vi "Start Sync.vi"(8 "error in (no error)":errorcluster, 10 "current time":timestamp, 11 "gRPC Server in":refnum<class "HVC2.lvclass">) -> (0 "error out":errorcluster, 3 "gRPC Server out":refnum<class "HVC2.lvclass">)   [LabVIEW 2019, in "HVC2.lvlib" / "HVC2.lvclass"]
uses:
  HVC2.lvclass
  RPC Messages/measurementservice_DMMConfigRequest/measurementservice_DMMConfigRequest_Data.ctl
  HVC2.lvclass/HVC2.ctl
  RPC Messages/measurementservice_QueryResponse/measurementservice_QueryResponse_Data.ctl
  RPC Messages/measurementservice_DMMConfigResponse/measurementservice_DMMConfigResponse_Data.ctl
  RPC Messages/measurementservice_ErrorOut/measurementservice_ErrorOut_Data.ctl
  RPC Messages/measurementservice_DMMVoltageData/measurementservice_DMMVoltageData_Data.ctl
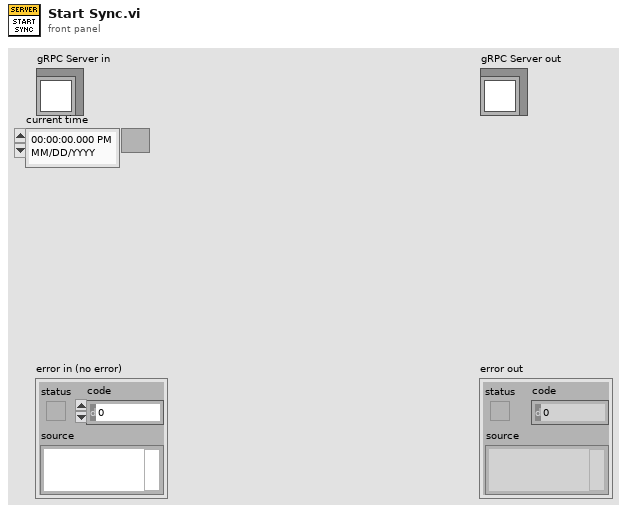
[diagram p1: front panel]
types:
  T1 = typedef "HVC2.lvlib/HVC2.lvclass/measurementservice_DMMConfigRequest_Data.ctl" = cluster{"DMMFunction":i32, "DMMResolution":sgl, "DMMRange":sgl, "DMMSampleCount":i32, "DMMApertureTimeUnit":i32, "DMMApertureTime":sgl, "DMMNumberofAverages":i32, "DMMAutoZero":i32, "DMMADCCalibration":i32, "DMMSettleTime":sgl}
  T2 = cluster{"measurementservice_DMMConfigRequest_Data":T1}
  T3 = typedef "HVC2.lvlib/HVC2.lvclass/measurementservice_QueryResponse_Data.ctl" = cluster{"message":string, "status":i32}
  T4 = typedef "HVC2.lvlib/HVC2.lvclass/measurementservice_ErrorOut_Data.ctl" = cluster{"errCode":i32, "errMessage":string}
  T5 = typedef "HVC2.lvlib/HVC2.lvclass/measurementservice_DMMConfigResponse_Data.ctl" = cluster{"DMMFunction":i32, "DMMResolution":sgl, "DMMRange":sgl, "DMMSampleCount":i32, "DMMApertureTimeUnit":i32, "DMMApertureTime":sgl, "DMMNumberofAverages":i32, "DMMAutoZero":i32, "DMMADCCalibration":i32, "DMMSettleTime":sgl, "error":T4}
  T6 = typedef "HVC2.lvlib/HVC2.lvclass/measurementservice_DMMVoltageData_Data.ctl" = cluster{"voltage":sgl, "error":T4}
  T7 = typedef "HVC2.lvlib/HVC2.lvclass/Server gRPC UEs.ctl" = cluster{"Invoke gRPC UE":refnum<user-event>, "Query gRPC UE":refnum<user-event>, "Register gRPC UE":refnum<user-event>, "ConfigureDMM gRPC UE":refnum<user-event>, "PerformDMMVoltageMeasurement gRPC UE":refnum<user-event>}
  T8 = typedef "HVC2.lvlib/gprc-lvsupport.lvlib/grpcId.ctl" = u64
  T9 = typedef "HVC2.lvlib/HVC2.lvclass/measurementservice_QueryRequest_Data.ctl" = cluster{"query":string}
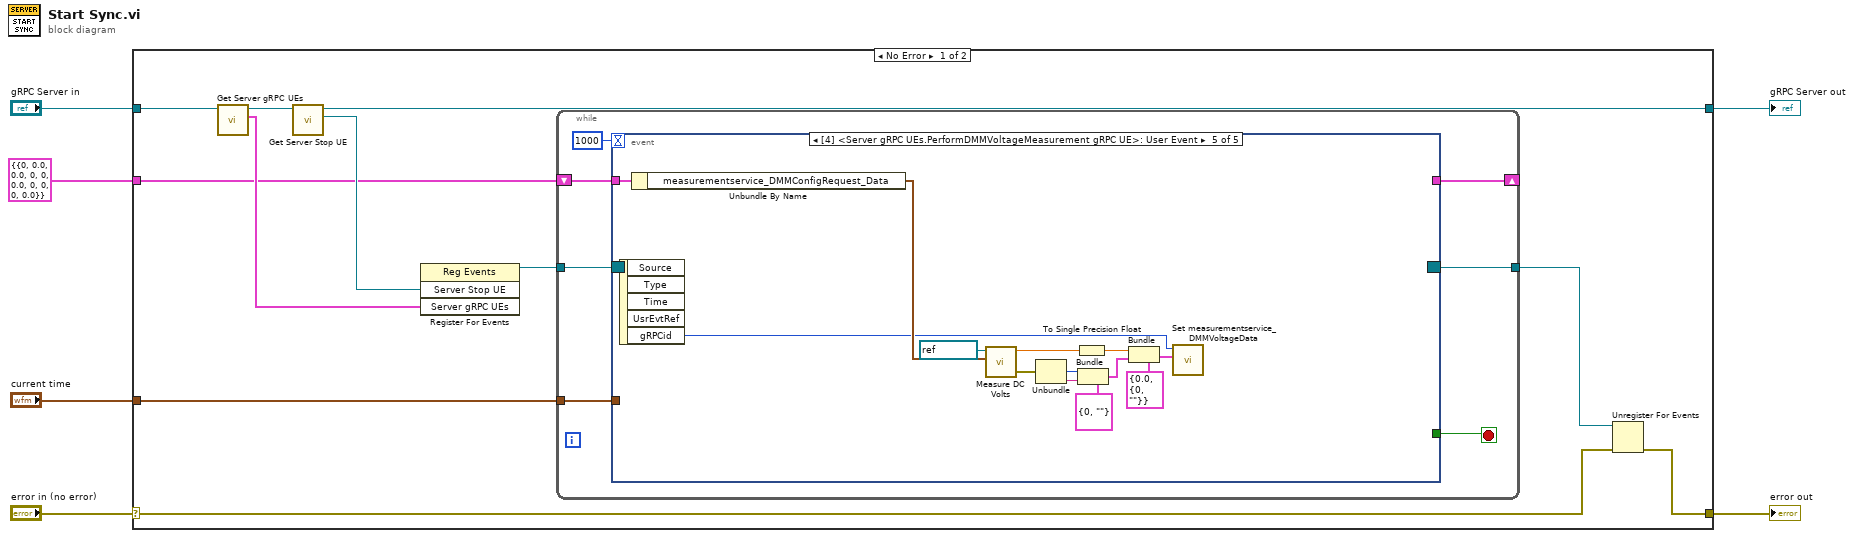
[diagram p0: block diagram]
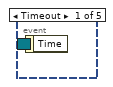
[diagram p2: hidden frame]
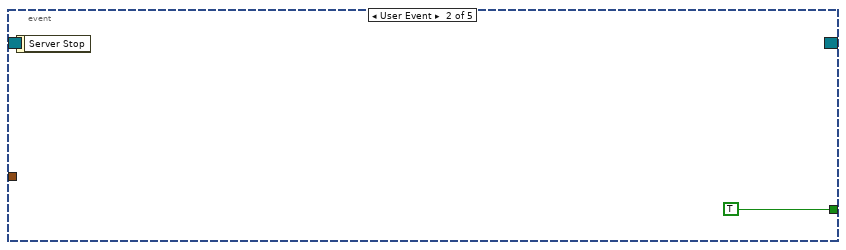
[diagram p3: hidden frame]
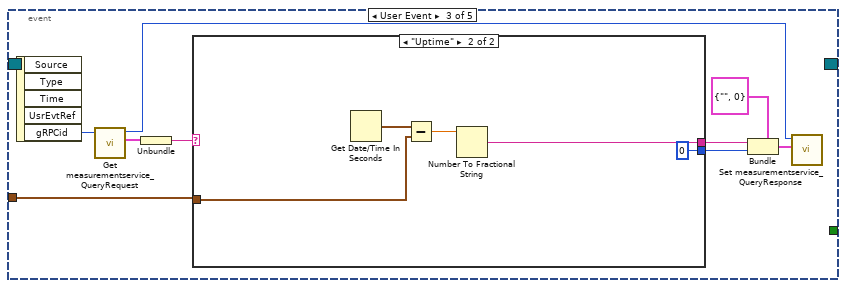
[diagram p4: hidden frame]
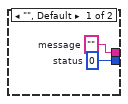
[diagram p5: hidden frame]
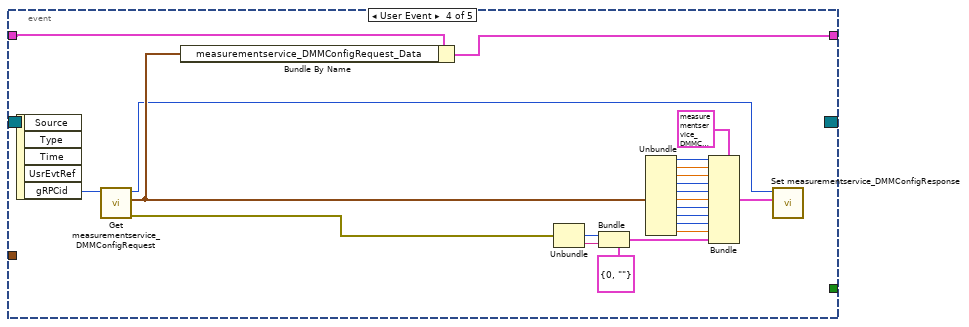
[diagram p6: hidden frame]
diagram:
  n1 = case shown="No Error" "error in (no error)" {
    selector: "error in (no error)" -> [w10 w78]
    tunnel: [w9 w78] -> w5
    tunnel: [w13 w77] -> w3
    tunnel: "gRPC Server in" -> [w17 w77]
    tunnel: "current time" -> [w8 _]
    tunnel: T2 {"measurementservice_DMMConfigRequest_Data"={"DMMFunction"=0, "DMMResolution"=0.0, "DMMRange"=0.0, "DMMSampleCount"=0, "DMMApertureTimeUnit"=0, "DMMApertureTime"=0.0, "DMMNumberofAverages"=0, "DMMAutoZero"=0, "DMMADCCalibration"=0, "DMMSettleTime"=0.0}} -> [w7 _]
    frame No Error {
      n2 = call "Get Server gRPC UEs.vi"("OOP Server in"=w17) -> ("Server gRPC UEs"=w14:T7, "OOP Server out"=w16:refnum<class "HVC2.lvclass">)  [unwired: 9 in]
      n3 = call "Get Server Stop UE.vi"("OOP Server in"=w16) -> ("Server Stop UE"=w15:refnum<user-event>, "OOP Server out"=w13:refnum<class "HVC2.lvclass">)  [unwired: 9 in]
      n4 = register-events(w15, w14) -> (reference out=w12:refnum<event-registration>)  [unwired: 2 in, 1 out]
      n5 = while {
        tunnel: w12 -> [w24]
        tunnel: [w22] -> w11
        tunnel: w8 -> [w20]
        shift-right: [w18] -> _
        shift-left: w7 -> [w19]
        stop <- w23 stop-if-true
        n6 = event "RPC Methods Event Structure" shown="[4] <Server gRPC UEs.PerformDMMVoltageMeasurement gRPC UE>: User Event" {
          selector: w24 -> [_ _ _ _ _]
          dyn-events: [_ _ _ _ _] -> w22
          timeout: 1000 -> [_ _ _ _ _]
          tunnel: [_ TRUE _ _ _] -> w23
          tunnel: w20 -> [_ _ w31 _ _]
          tunnel: w19 -> [_ _ _ w61 w76]
          tunnel: [_ _ _ w60 _] -> w18
          event Timeout {
            n7 = event-data() -> ()  [unwired: 1 in, 1 out]
          }
          event User Event {
            n8 = event-data() -> ()  [unwired: 1 in, 1 out]
          }
          event User Event {
            n9 = event-data() -> ("gRPCid"=w30:T8)  [unwired: 1 in, 4 out]
            n10 = call "Get measurementservice_QueryRequest.vi"("gRPCid"=w30) -> ("Message Data"=w29:T9, "gRPCid out"=w27:T8)  [unwired: 8 in, 1 out]
            n11 = Unbundle(w29) -> ("query"=w34:string)
            n12 = case shown="\"Uptime\"" w34 {
              tunnel: [w36 0 ("status")] -> w33
              tunnel: [w35 w38] -> w32
              tunnel: w31 -> [_ w40]
              frame "", Default {
                w35 = ""  # message
                w36 = 0  # status
              }
              frame "Uptime" {
                n13 = Get Date/Time In Seconds() -> (seconds since 1Jan1904=w41:timestamp)
                n14 = Subtract(x=w41, y=w40) -> (x-y=w39:dbl)
                n15 = Number To Fractional String(number=w39) -> (F-format string=w38:string)  [unwired: 3 in]
              }
            }
            n16 = Bundle(cluster=T3 {"message"="", "status"=0} ("measurementservice_QueryResponse_Data"), "message"=w32, "status"=w33) -> (w26:T3)
            n17 = call "Set measurementservice_QueryResponse.vi"("Message Data"=w26, "gRPCid"=w27) -> ()  [unwired: 9 in, 1 out]
          }
          event User Event {
            n18 = event-data() -> ("gRPCid"=w63:T8)  [unwired: 1 in, 4 out]
            n19 = call "Get measurementservice_DMMConfigRequest.vi"("gRPCid"=w63) -> ("error out"=w46:errorcluster, "Message Data"=w62:T1, "gRPCid out"=w57:T8)  [unwired: 8 in]
            n20 = Bundle By Name(cluster=w61, "measurementservice_DMMConfigRequest_Data"=w62) -> (w60:T2)
            n21 = Unbundle(w46) -> ("code"=w44:i32, "source"=w43:string)  [unwired: 1 out]
            n22 = Bundle(cluster=T4 {"errCode"=0, "errMessage"=""} ("error"), "errCode"=w44, "errMessage"=w43) -> (w42:T4)
            n23 = Unbundle(w62) -> ("DMMFunction"=w56:i32, "DMMResolution"=w55:sgl, "DMMRange"=w54:sgl, "DMMSampleCount"=w53:i32, "DMMApertureTimeUnit"=w52:i32, "DMMApertureTime"=w51:sgl, "DMMNumberofAverages"=w50:i32, "DMMAutoZero"=w49:i32, "DMMADCCalibration"=w48:i32, "DMMSettleTime"=w47:sgl)
            n24 = Bundle(cluster=T5 {"DMMFunction"=0, "DMMResolution"=0.0, "DMMRange"=0.0, "DMMSampleCount"=0, "DMMApertureTimeUnit"=0, "DMMApertureTime"=0.0, "DMMNumberofAverages"=0, "DMMAutoZero"=0, "DMMADCCalibration"=0, "DMMSettleTime"=0.0, "error"={"errCode"=0, "errMessage"=""}} ("measurementservice_DMMConfigResponse_Data"), "DMMFunction"=w56, "DMMResolution"=w55, "DMMRange"=w54, "DMMSampleCount"=w53, "DMMApertureTimeUnit"=w52, "DMMApertureTime"=w51, "DMMNumberofAverages"=w50, "DMMAutoZero"=w49, "DMMADCCalibration"=w48, "DMMSettleTime"=w47, "error"=w42) -> (w58:T5)
            n25 = call "Set measurementservice_DMMConfigResponse.vi"("Message Data"=w58, "gRPCid"=w57) -> ()  [unwired: 9 in, 1 out]
          }
          event User Event {
            n26 = event-data() -> ("gRPCid"=w64:T8)  [unwired: 1 in, 4 out]
            n27 = Unbundle By Name(w76) -> ("measurementservice_DMMConfigRequest_Data"=w74:T1)
            n28 = call "Measure DC Volts.vi"("measurementservice_DMMConfigRequest_Data"=w74, "IVI Refnum in"=refnum<k15> "DMM" ("Device Name")) -> ("error out"=w70:errorcluster, "Measurement (Volts)"=w72:dbl)  [unwired: 8 in]
            n29 = Unbundle(w70) -> ("code"=w68:i32, "source"=w67:string)  [unwired: 1 out]
            n30 = To Single Precision Float(number=w72) -> (single precision float=w71:sgl)
            n31 = Bundle(cluster=T4 {"errCode"=0, "errMessage"=""} ("error"), "errCode"=w68, "errMessage"=w67) -> (w66:T4)
            n32 = Bundle(cluster=T6 {"voltage"=0.0, "error"={"errCode"=0, "errMessage"=""}} ("measurementservice_DMMVoltageData_Data"), "voltage"=w71, "error"=w66) -> (w65:T6)
            n33 = call "Set measurementservice_DMMVoltageData.vi"("Message Data"=w65, "gRPCid"=w64) -> ()  [unwired: 9 in, 1 out]
          }
        }
      }
      n34 = Unregister For Events(event registration refnum=w11, error in=w10) -> (error out=w9:errorcluster)
    }
    frame Error {
    }
  }
  "error out" <- w5
  "gRPC Server out" <- w3
